vi "Close.vi"(8 "error in (no error)":errorcluster) -> (0 "error out":errorcluster)   [LabVIEW 2009, in "Main.lvlib"]
doc: "Main Close VI, executes on shutdown of the main program. Closes all references in the program."
uses:
  Main.lvlib
  OWNCAN.lvlib
  FPGA.lvlib
  ImageProject/Camera.lvlib
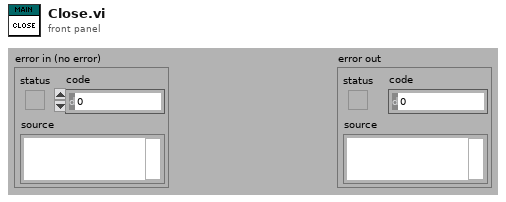
[diagram p1: front panel]
types:
  T1 = typedef "Semaphore RefNum" = refnum<k1>
  T2 = cluster{"CAN Jaguar Ref Left":cluster{"Device Number":u8, "Control Mode":enum16{"Percent VBus", "Speed", "Position", "Current"}, "Inverted":bool, "Semaphore":T1, "Max Vout":dbl, "DevStatus":errorcluster}, "CAN Jaguar Ref Right":cluster{"Device Number":u8, "Control Mode":enum16{"Percent VBus", "Speed", "Position", "Current"}, "Inverted":bool, "Semaphore":T1, "Max Vout":dbl, "DevStatus":errorcluster}}
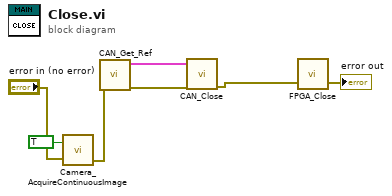
[diagram p0: block diagram]
diagram:
  n1 = call "Camera_AcquireContinuousImage.vi"("Stop (F)"=TRUE, "error in"="error in (no error)") -> ("error out"=w2:errorcluster)  [unwired: 2 out]
  n2 = call "CAN_Get_Ref.vi"("error in (no error)"=w2) -> ("error out"=w6:errorcluster, "CAN_Jaguars_ref"=w7:T2)  [unwired: 9 in]
  n3 = call "CAN_Close.vi"("error in"=w6, "CAN Jaguars Ref"=w7) -> ("error out"=w5:errorcluster)  [unwired: 9 in]
  n4 = call "FPGA_Close.vi"("error in (no error)"=w5) -> ("error out"=→"error out":errorcluster)  [unwired: 2 in]
